vi "RubikStart.vi"   [LabVIEW 2017]
uses:
  Projekt-RubikLibrary/ServoAbsAngleControl.ctl
  Projekt-RubikLibrary/ServoEnumControl.ctl
  Projekt-RubikLibrary/RubikLibrary.lvlib
types:
  T1 = typedef "RubikLibrary.lvlib/ServoEnumControl.ctl" = enum16{"Left Servo", "Front Servo", "Right Servo"}
  T2 = typedef "RubikLibrary.lvlib/ServoAbsAngleControl.ctl" = i16
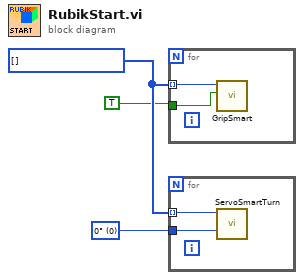
[diagram p0: block diagram]
diagram:
  w3 = T1[] [] items=["Left Servo", "Front Servo", "Right Servo"] ("Array")
  w2 = T2 0 items=["-90°"=-90, "0°"=0, "+90°"=90] ("Turn to")
  n1 = for {
    tunnel: w3 -> [w5] mode=indexing
    tunnel: TRUE -> [w4]
    n2 = call "GripSmart.vi"("Turn to (in)"=w4, "Servo"=w5) -> ()  [unwired: 8 in, 2 out]
  }
  n3 = for {
    tunnel: w3 -> [w7] mode=indexing
    tunnel: w2 -> [w6]
    n4 = call "ServoSmartTurn.vi"("Turn to (in)"=w6, "Servo"=w7) -> ()  [unwired: 8 in, 2 out]
  }
